vi "Fetch Child Libraries.vi"(8 "Error in":errorcluster caption="Error in (no error)", 11 "Library in":refnum<vi>) -> (0 "Error out":errorcluster, 2 "Child Libraries":T1[](array[typedef]), 3 "Library out":refnum<vi>)   [LabVIEW 2023, in "VIDoc Parsing.lvlib" / "Library Documentation.lvclass"]
uses:
  Library Documentation.lvclass
  Child Libraries Cluster.ctl
  Library Documentation.lvclass/Library Documentation.ctl
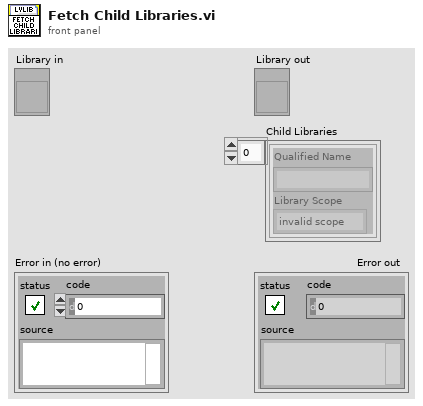
[diagram p1: front panel]
types:
  T1 = typedef "VIDoc Parsing.lvlib/Library Documentation.lvclass/Child Libraries Cluster.ctl" = cluster{"Qualified Name":string, "Library Scope":enum32{"invalid scope", "public", "private", "protected", "community"}}
  T2 = enum32{"invalid scope", "public", "private", "protected", "community"}
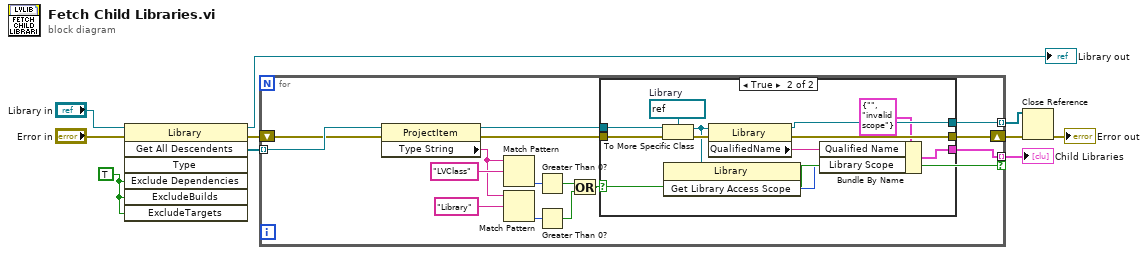
[diagram p0: block diagram]
diagram:
  w10 = TRUE ("ExcludeDependencies")
  n1 = invoke class="Library" method="Get All Descendents"(reference="Library in", error in="Error in", "Exclude Dependencies"=w10, "ExcludeBuilds"=w10, "ExcludeTargets"=w10) -> (reference out=→"Library out":refnum<vi>, error out=w7:errorcluster, "All Descendents"=w9:refnum<vi>[])  [unwired: 2 in, 4 out]
  n2 = for {
    tunnel: w9 -> [w25] mode=indexing
    tunnel: [w20] -> w8 mode=indexing
    tunnel: [w19] -> w1 mode=indexing if=w16
    shift-right: [w21] -> w6
    shift-left: w7 -> [w24]
    n3 = property class="ProjectItem"(reference=w25, error in=w24) -> (reference out=w22:refnum<vi>, error out=w23:errorcluster, "Type String"=w12:string)
    n4 = Match Pattern(string=w12, regular expression="LVClass" ("String")) -> (offset past match=w18:i32)  [unwired: 4 out]
    n5 = Match Pattern(string=w12, regular expression="Library" ("String")) -> (offset past match=w14:i32)  [unwired: 4 out]
    n6 = Greater Than 0?(x=w18) -> (x > 0?=w17:bool)
    n7 = Greater Than 0?(x=w14) -> (x > 0?=w11:bool)
    n8 = Or(x=w17, y=w11) -> (x .or. y?=w16:bool)
    n9 = case shown="True" w16 {
      tunnel: w23 -> [w26 w38]
      tunnel: w22 -> [w27 w36]
      tunnel: [w26 w34] -> w21
      tunnel: [w27 w33] -> w20
      tunnel: [_ w31] -> w19
      frame False {
      }
      frame True {
        w35 = refnum<vi> refnum  # Library
        n10 = To More Specific Class(target class=w35, reference=w36, error in=w38) -> (specific class reference=w29:refnum<vi>, error out=w37:errorcluster)
        n11 = invoke class="Library" method="Get Library Access Scope"(reference=w29) -> ("Get Library Access Scope"=w28:T2)  [unwired: 2 in, 2 out]
        n12 = property class="Library"(reference=w29, error in=w37) -> (reference out=w33:refnum<vi>, error out=w34:errorcluster, "QualifiedName"=w30:string)
        n13 = Bundle By Name(cluster=T1 {"Qualified Name"="", "Library Scope"=enum."invalid scope"} ("Child Library"), "Qualified Name"=w30, "Library Scope"=w28) -> (w31:T1)
      }
    }
  }
  "Child Libraries" <- w1
  n14 = Close Reference(reference=w8, error in (no error)=w6) -> (error out=→"Error out":errorcluster)
